vi "Main.vi"(8 "error in":errorcluster, 11 "GraphUI in":refnum<class "GraphUI.lvclass">) -> (0 "error out":errorcluster, 3 "GraphUI out":refnum<class "GraphUI.lvclass">)   [LabVIEW 2023, in "GraphUI.lvclass"]
doc: "The <b>Queued Message Handler</b> of the Worker that owns this VI."
uses:
  GraphUI.lvclass
  C:/Program Files/National Instruments/LabVIEW 2023/vi.lib/addons/_Workers/Library/Classes/Worker/Worker.lvclass
  Initialization Data.ctl
  Response Cases.ctl
  GraphUI.lvclass/GraphUI.ctl
  <vilib>/addons/_Workers/Library/Classes/Message Queue/Message Queue.lvclass
panel:
  out "Graph Name":string
  in  "Pause Tool":bool
  out "График":dbl(graph) caption="Waveform Chart - Dark"
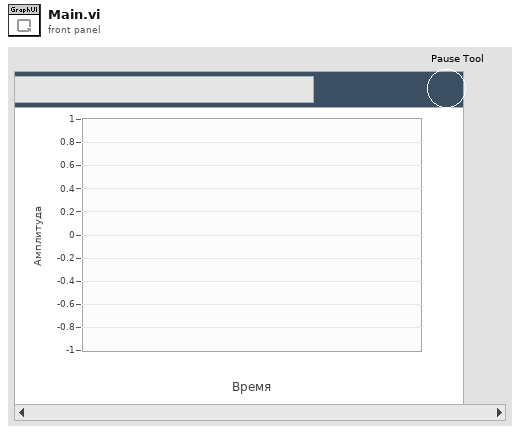
[diagram p1: front panel]
types:
  T1 = typedef "GraphUI.lvclass/Initialization Data.ctl" = cluster{"Response Cases":T2, "Control ref":refnum<vi>}
  T2 = typedef "GraphUI.lvclass/Response Cases.ctl" = cluster{"Placeholder - Can be deleted":string}
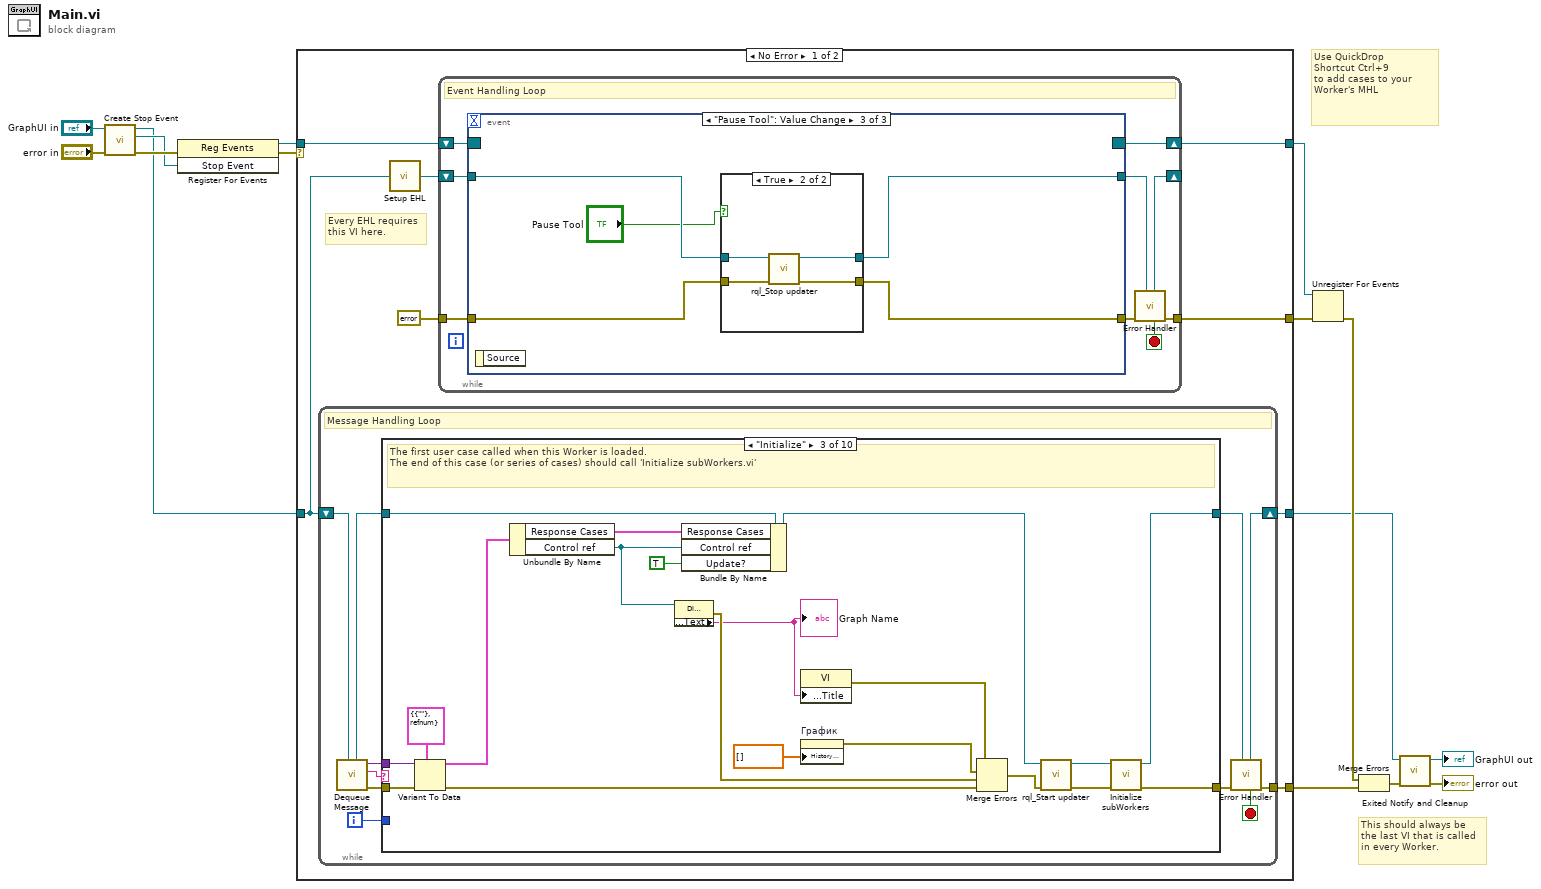
[diagram p0: block diagram]
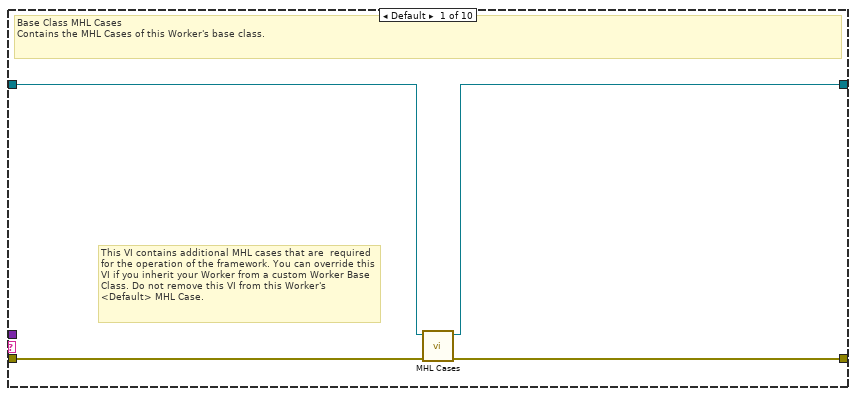
[diagram p2: hidden frame]
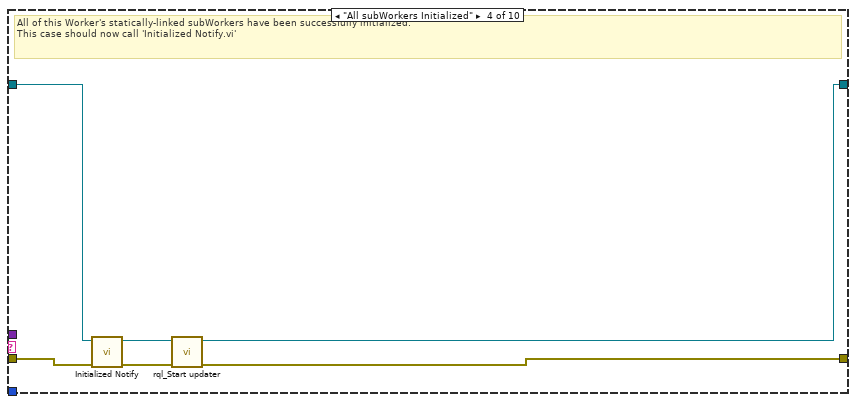
[diagram p4: hidden frame]
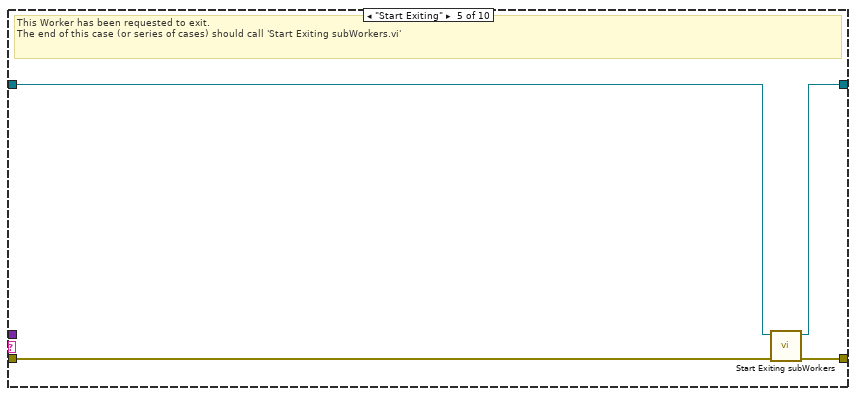
[diagram p5: hidden frame]
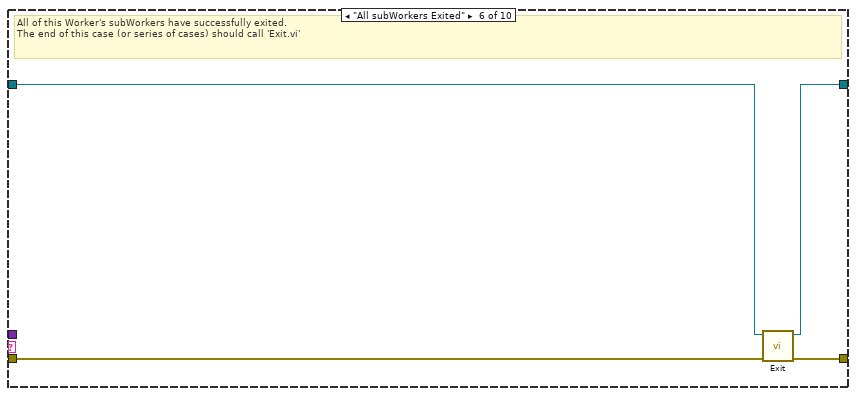
[diagram p6: hidden frame]
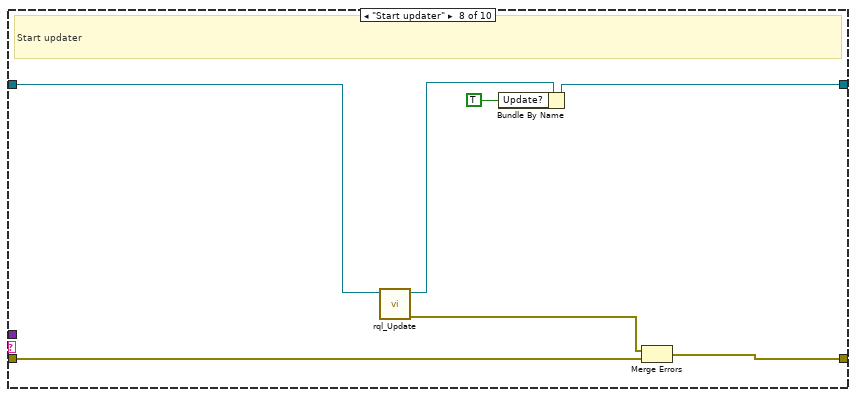
[diagram p8: hidden frame]
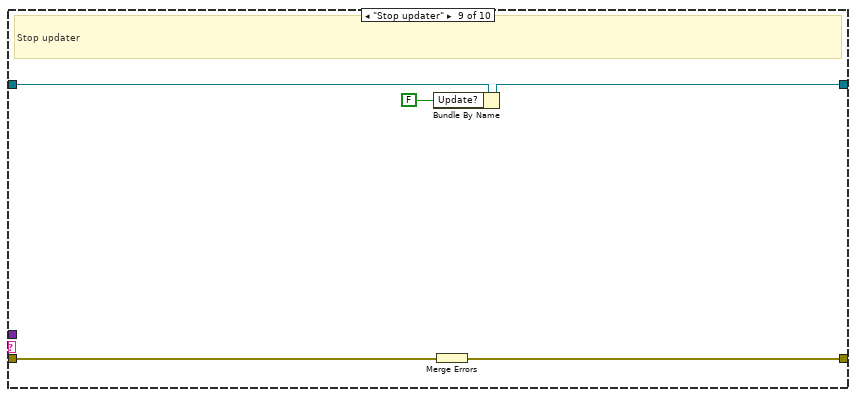
[diagram p9: hidden frame]
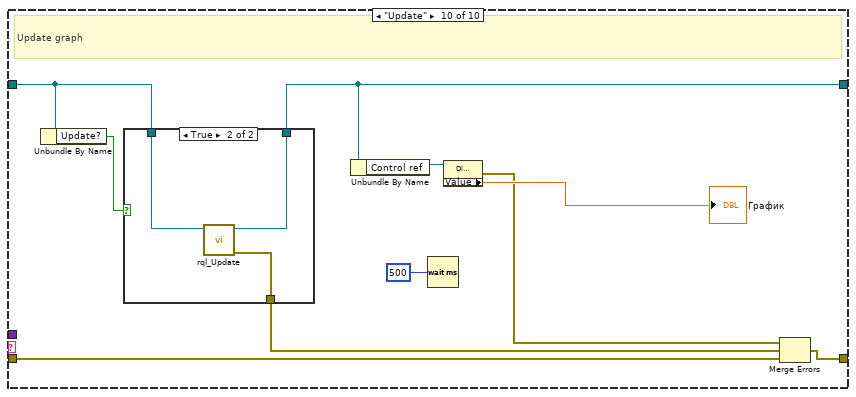
[diagram p10: hidden frame]
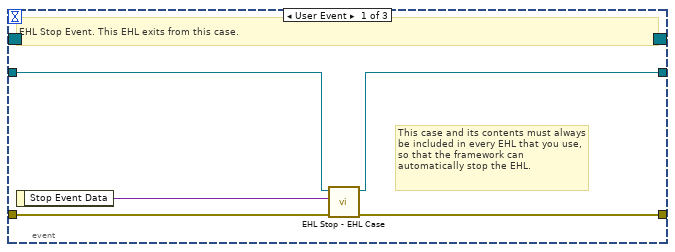
[diagram p12: hidden frame]
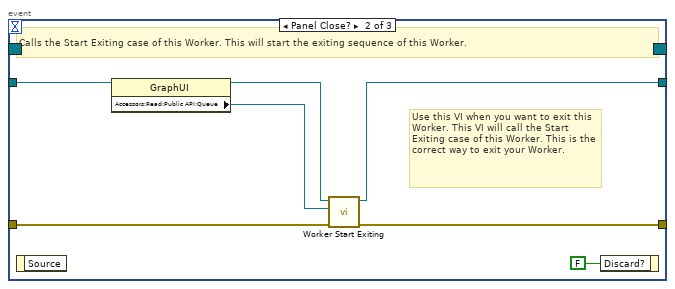
[diagram p13: hidden frame]
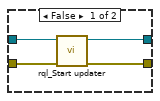
[diagram p14: hidden frame]
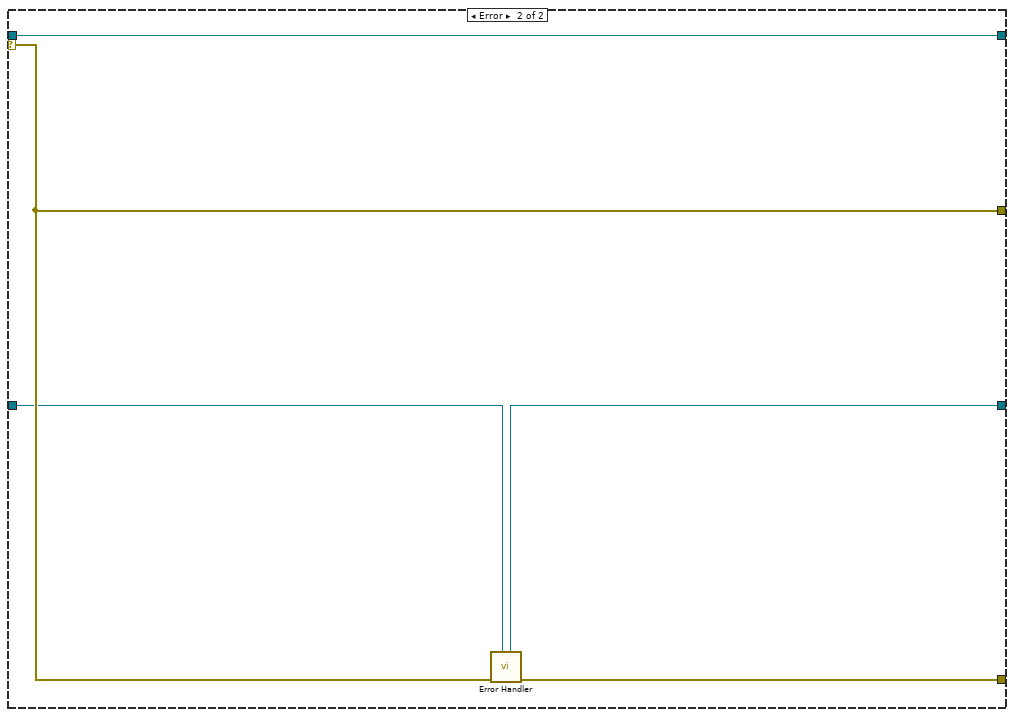
[diagram p15: hidden frame]
diagram:
  # "Use QuickDrop\nShortcut Ctrl+9\nto add cases to your\nWorker's MHL"
  # "This should always be the last VI that is called in every Worker."
  n1 = call-dynamic "Create Stop Event.vi"("error in"="error in", "Worker"="GraphUI in") -> ("error out"=w10:errorcluster, "Stop Event"=w7:refnum<user-event>, "Worker out"=w4:refnum<class "GraphUI.lvclass">)  [unwired: 7 in]
  n2 = register-events(error in=w10, w7) -> (reference out=w9:refnum<event-registration>, error out=w1:errorcluster)  [unwired: 1 in]
  n3 = case shown="No Error" w1 {
    tunnel: w4 -> [w18 w138]
    tunnel: [w16 w139] -> w8
    tunnel: w9 -> [w23 w140]
    tunnel: [w20 w141] -> w14
    tunnel: [w22 w140] -> w13
    tunnel: [w17 w137] -> w11
    selector: w1 -> [_ w141]
    frame No Error {
      # "Every EHL requires\nthis VI here."
      n4 = while {
        shift-right: [w32] -> w17
        shift-left: w18 -> [w34]
        tunnel: [w33] -> w16
        i -> [w25]
        stop <- w26 stop-if-true
        # "Message Handling Loop"
        n5 = call-dynamic "Dequeue Message.vi"("Worker"=w34) -> ("error out"=w31:errorcluster, "Case out"=w27:string, "Data out"=w24:variant, "Worker out"=w29:refnum<class "GraphUI.lvclass">)  [unwired: 6 in, 1 out]
        n6 = case "Worker MHL Case Structure (DO NOT CHANGE LABEL NAME)" shown="\"Initialize\"" w27 {
          tunnel: w31 -> [w38 w39 w58 w65 w67 w74 w76 w77 w84 w90]
          tunnel: [w37 w39 w60 w62 w70 w73 w76 w83 w87 w98] -> w30
          tunnel: w29 -> [w36 w40 w57 w66 w68 w72 w75 w80 w88 w95]
          tunnel: [w35 w40 w59 w61 w69 w71 w75 w82 w86 w94] -> w28
          tunnel: w25 -> [_ _ _ _ _ _ _ _ _ _]
          tunnel: w24 -> [_ _ w55 _ _ _ _ _ _ _]
          frame Default {
            # "This VI contains additional MHL cases that are  required for the operation of the framework. You can override this VI if you inherit your Worker from a custom Worker Base Class. Do not remove this VI from this Worker's <Default> MHL Case."
            # "Base Class MHL Cases\nContains the MHL Cases of this Worker's base class."
            n7 = call-dynamic "MHL Cases.vi"("error in"=w38, "Worker in"=w36) -> ("error out"=w37:errorcluster, "Worker out"=w35:refnum<class "GraphUI.lvclass">)  [unwired: 8 in]
          }
          frame "------------ FRAMEWORK CASES -----------" {
            # "Start of Workers Framework Cases"
          }
          frame "Initialize" {
            # "The first user case called when this Worker is loaded.\nThe end of this case (or series of cases) should call 'Initialize subWorkers.vi'"
            n8 = Variant To Data(error in=w58, type=T1 {"Response Cases"={"Placeholder - Can be deleted"=""}, "Control ref"=refnum} ("Initialization Data"), Variant=w55) -> (data=w54:T1, error out=w56:errorcluster)
            n9 = Unbundle By Name(w54) -> ("Response Cases"=w53:T2, "Control ref"=w46:refnum<vi>)
            n10 = property class="DigNum (strict)"(reference=w46) -> (error out=w45:errorcluster, "Caption.Text"=w42:string)  [unwired: 1 in, 1 out]
            "Graph Name" <- w42
            n11 = Bundle By Name(cluster=w57, "Response Cases"=w53, "Control ref"=w46, "Update?"=TRUE) -> (w50:refnum<class "GraphUI.lvclass">)
            n12 = property class="VI"("Front Panel.Title"=w42) -> (error out=w41:errorcluster)  [unwired: 2 in, 1 out]
            n13 = property on="График" class="WFChart (strict)"("History Data"=dbl[] []) -> (error out=w43:errorcluster)  [unwired: 2 in, 1 out]
            n14 = Merge Errors(w41, w43, w45, w56) -> (w47:errorcluster)
            n15 = call "rql_Start updater.vi"("error in"=w47, "GraphUI in"=w50) -> ("error out"=w48:errorcluster, "dup GraphUI out"=w49:refnum<class "GraphUI.lvclass">)  [unwired: 8 in]
            n16 = call-dynamic "Initialize subWorkers.vi"("error in"=w48, "Worker"=w49) -> ("error out"=w60:errorcluster, "dup Worker out"=w59:refnum<class "GraphUI.lvclass">)  [unwired: 8 in]
          }
          frame "All subWorkers Initialized" {
            # "All of this Worker's statically-linked subWorkers have been successfully initialized.\nThis case should now call 'Initialized Notify.vi'"
            n17 = call-dynamic "Initialized Notify.vi"("error in"=w65, "Worker"=w66) -> ("error out"=w64:errorcluster, "dup Worker out"=w63:refnum<class "GraphUI.lvclass">)  [unwired: 8 in]
            n18 = call "rql_Start updater.vi"("error in"=w64, "GraphUI in"=w63) -> ("error out"=w62:errorcluster, "dup GraphUI out"=w61:refnum<class "GraphUI.lvclass">)  [unwired: 8 in]
          }
          frame "Start Exiting" {
            # "This Worker has been requested to exit. \nThe end of this case (or series of cases) should call 'Start Exiting subWorkers.vi'"
            n19 = call-dynamic "Start Exiting subWorkers.vi"("error_in"=w67, "Worker"=w68) -> ("error out"=w70:errorcluster, "dup Worker out"=w69:refnum<class "GraphUI.lvclass">)  [unwired: 8 in]
          }
          frame "All subWorkers Exited" {
            # "All of this Worker's subWorkers have successfully exited. \nThe end of this case (or series of cases) should call 'Exit.vi'"
            n20 = call-dynamic "Exit.vi"("error_in"=w74, "Worker"=w72) -> ("error out"=w73:errorcluster, "dup Worker out"=w71:refnum<class "GraphUI.lvclass">)  [unwired: 8 in]
          }
          frame "------------- LOCAL API CASES -------------" {
            # "Start of Workers Local API Cases"
          }
          frame "Start updater" {
            # "Start updater"
            n21 = call "rql_Update.vi"("GraphUI in"=w80) -> ("error out"=w78:errorcluster, "dup GraphUI out"=w79:refnum<class "GraphUI.lvclass">)  [unwired: 9 in]
            n22 = Bundle By Name(cluster=w79, "Update?"=TRUE) -> (w82:refnum<class "GraphUI.lvclass">)
            n23 = Merge Errors(w78, w77) -> (w83:errorcluster)
          }
          frame "Stop updater" {
            # "Stop updater"
            n24 = Bundle By Name(cluster=w88, "Update?"=FALSE) -> (w86:refnum<class "GraphUI.lvclass">)
            n25 = Merge Errors(w84) -> (w87:errorcluster)
          }
          frame "Update" {
            # "Update graph"
            n26 = Unbundle By Name(w95) -> ("Update?"=w96:bool)
            n27 = case shown="True" w96 {
              tunnel: [_ w102] -> w97
              tunnel: w95 -> [w99 w101]
              tunnel: [w99 w100] -> w94
              frame False {
              }
              frame True {
                n28 = call "rql_Update.vi"("GraphUI in"=w101) -> ("error out"=w102:errorcluster, "dup GraphUI out"=w100:refnum<class "GraphUI.lvclass">)  [unwired: 9 in]
              }
            }
            n29 = Unbundle By Name(w94) -> ("Control ref"=w93:refnum<vi>)
            n30 = Wait (ms)(milliseconds to wait=u32 500) -> ()  [unwired: 1 out]
            n31 = property class="DigNum (strict)"(reference=w93) -> (error out=w89:errorcluster, "Value"=→"График":dbl)  [unwired: 1 in, 1 out]
            n32 = Merge Errors(w89, w97, w90) -> (w98:errorcluster)
          }
        }
        n33 = call-dynamic "Error Handler.vi"("Worker"=w28, "error_in"=w30) -> ("error out"=w33:errorcluster, "Stop Loop"=w26:bool, "Worker out"=w32:refnum<class "GraphUI.lvclass">)  [unwired: 7 in]
      }
      n34 = call-dynamic "Setup EHL.vi"("Worker"=w18) -> ("Worker out"=w19:refnum<class "GraphUI.lvclass">)  [unwired: 14 in]
      n35 = while "Event Handling Loop" {
        shift-right: [w111] -> w22
        shift-left: w23 -> [w110]
        tunnel: [w106] -> w20
        tunnel: errorcluster {"status"=FALSE, "code"=0, "source"=""} ("error constant") -> [w108]
        shift-right: [w104] -> _
        shift-left: w19 -> [w109]
        stop <- w103 stop-if-true
        # "Event Handling Loop"
        n36 = event shown="[2] \"Pause Tool\": Value Change" {
          selector: w110 -> [_ _ _]
          dyn-events: [_ _ _] -> w111
          timeout: _ -> [_ _ _]
          tunnel: [w115 w122 w125] -> w107
          tunnel: w108 -> [w116 w121 w126]
          tunnel: w109 -> [w114 w120 w128]
          tunnel: [w113 w119 w127] -> w105
          event User Event {
            # "This case and its contents must always be included in every EHL that you use, so that the framework can automatically stop the EHL."
            # "EHL Stop Event. This EHL exits from this case."
            n37 = event-data() -> ("Stop Event Data"=w112:variant)  [unwired: 1 in]
            n38 = call-dynamic "EHL Stop - EHL Case.vi"("error in"=w116, "Stop Event Data"=w112, "Worker"=w114) -> ("error out"=w115:errorcluster, "Worker out"=w113:refnum<class "GraphUI.lvclass">)  [unwired: 7 in]
          }
          event Panel Close? {
            # "Use this VI when you want to exit this Worker. This VI will call the Start Exiting case of this Worker. This is the correct way to exit your Worker."
            # "Calls the Start Exiting case of this Worker. This will start the exiting sequence of this Worker."
            n39 = event-data() -> ()  [unwired: 1 in, 1 out]
            n40 = property class="GraphUI"(reference=w120) -> (reference out=w118:refnum<class "GraphUI.lvclass">, "Accessors:Read:Public API:Queue"=w117:refnum<class "Message Queue.lvclass">)  [unwired: 1 in, 1 out]
            n41 = call-dynamic "Worker Start Exiting.vi"("error_in"=w121, "Message Queue"=w117, "Worker"=w118) -> ("error out"=w122:errorcluster, "dup Worker out"=w119:refnum<class "GraphUI.lvclass">)  [unwired: 7 in]
            n42 = event-data("Discard?"=FALSE) -> ()  [unwired: 1 in, 1 out]
          }
          event "Pause Tool": Value Change {
            n43 = event-data() -> ()  [unwired: 1 in, 1 out]
            n44 = case shown="True" "Pause Tool" {
              tunnel: w128 -> [w132 w134]
              tunnel: [w131 w135] -> w127
              tunnel: w126 -> [w130 w133]
              tunnel: [w129 w136] -> w125
              frame False {
                n45 = call "rql_Start updater.vi"("error in"=w130, "GraphUI in"=w132) -> ("error out"=w129:errorcluster, "dup GraphUI out"=w131:refnum<class "GraphUI.lvclass">)  [unwired: 8 in]
              }
              frame True {
                n46 = call "rql_Stop updater.vi"("error in"=w133, "GraphUI in"=w134) -> ("error out"=w136:errorcluster, "dup GraphUI out"=w135:refnum<class "GraphUI.lvclass">)  [unwired: 8 in]
              }
            }
          }
        }
        n47 = call-dynamic "Error Handler.vi"("Worker"=w105, "error_in"=w107) -> ("error out"=w106:errorcluster, "Stop Loop"=w103:bool, "Worker out"=w104:refnum<class "GraphUI.lvclass">)  [unwired: 7 in]
      }
    }
    frame Error {
      n48 = call-dynamic "Error Handler.vi"("Worker"=w138, "error_in"=w141) -> ("error out"=w139:errorcluster, "Worker out"=w137:refnum<class "GraphUI.lvclass">)  [unwired: 7 in, 1 out]
    }
  }
  n49 = Unregister For Events(event registration refnum=w13, error in=w14) -> (error out=w15:errorcluster)
  n50 = Merge Errors(w15, w8) -> (w12:errorcluster)
  n51 = call-dynamic "Exited Notify and Cleanup.vi"("error_in"=w12, "Worker"=w11) -> ("error out"=→"error out":errorcluster, "dup Worker out"=→"GraphUI out":refnum<class "GraphUI.lvclass">)  [unwired: 8 in]
